vi "Reset.vi"(8 "error in (no error)":errorcluster, 11 "RP Transceiver in":refnum<class "RP Transceiver.lvclass">) -> (0 "error out":errorcluster, 3 "RP Transceiver out":refnum<class "RP Transceiver.lvclass">)   [LabVIEW 2015, in "RP Transceiver.lvclass"]
uses:
  RP Transceiver.lvclass
  RP Command.ctl
  RP Transceiver.lvclass/RP Transceiver.ctl
  RP Communicator/RP Communicator.lvclass
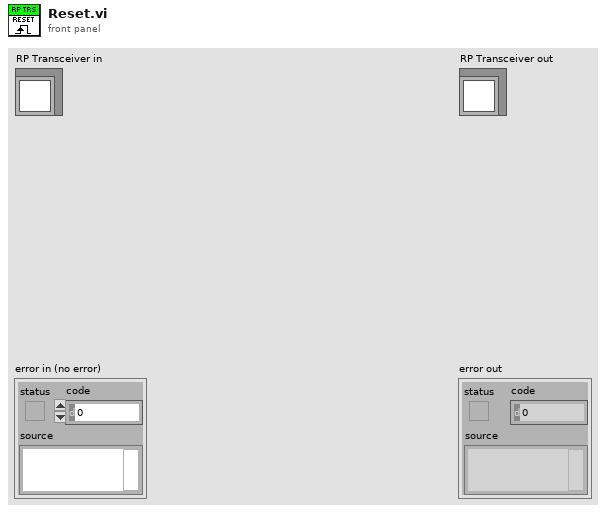
[diagram p1: front panel]
types:
  T1 = typedef "RP Command.ctl" = enum16{"Reset", "Read IDN", "Stop server", "Get status", "Get temperature", "Connect client", "Arm", "Software trigger", "Get whole buffer", "Get chunk", "System call", "Get config", "Set config", "Recieve data", "Play pattern", "Transmit data"}
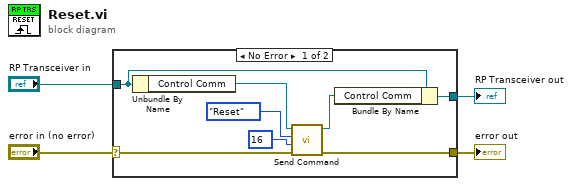
[diagram p0: block diagram]
diagram:
  n1 = case shown="No Error" "error in (no error)" {
    selector: "error in (no error)" -> [w6 w14]
    tunnel: [w5 w14] -> w3
    tunnel: [w9 w13] -> w1
    tunnel: "RP Transceiver in" -> [w10 w13]
    frame No Error {
      n2 = Unbundle By Name(w10) -> ("Control Comm"=w7:refnum<class "RP Communicator.lvclass">)
      n3 = call-dynamic "Send Command.vi"("error in (no error)"=w6, "Command payload"=u64 16, "Command number"=RP_Command."Reset", "RP Communicator in"=w7) -> ("error out"=w5:errorcluster, "RP Communicator out"=w8:refnum<class "RP Communicator.lvclass">)  [unwired: 6 in]
      n4 = Bundle By Name(cluster=w10, "Control Comm"=w8) -> (w9:refnum<class "RP Transceiver.lvclass">)
    }
    frame Error {
    }
  }
  "error out" <- w3
  "RP Transceiver out" <- w1
